vi "NF WF1973_74 TRAC Copy.vi"(5 "Name(USERNAME)":string="USERNAME", 7 "Memory No.(0)":i32 min=0 max=128 step=1, 8 "error in (no error)":errorcluster caption="Error IN", 9 "Select Function(Sin)":i32(ring)=2 items=["Sinusoid", "Square", "Pulse", "Ramp", "USine", "CSine", "CFCSine", "ACSine", "SSine", "MCSine", "ONPSine", "OFPSine", "CONSine", "COFSine", "Gaussian", "Lorents", "Haversine", "HSPulse", "TPulse", "Sinc", "ERise", "EFall", "Solstep", "Doscillation", "OSurge", "PSurge", "TOffset", "HSEPulse", "BRRamp", "USER"], 10 "Ch?(Ch1)":bool, 11 "VISAsession":refnum<visa-resource-name>) -> (0 "error out":errorcluster caption="Error OUT", 3 "CopyVISAsession":refnum<visa-resource-name>)   [LabVIEW 2010]
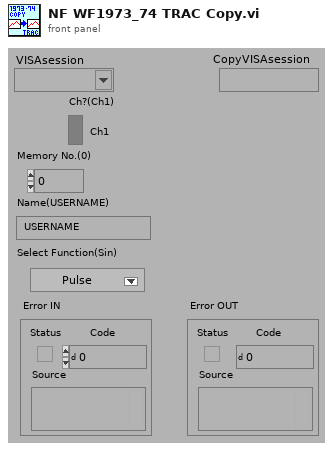
[diagram p1: front panel]
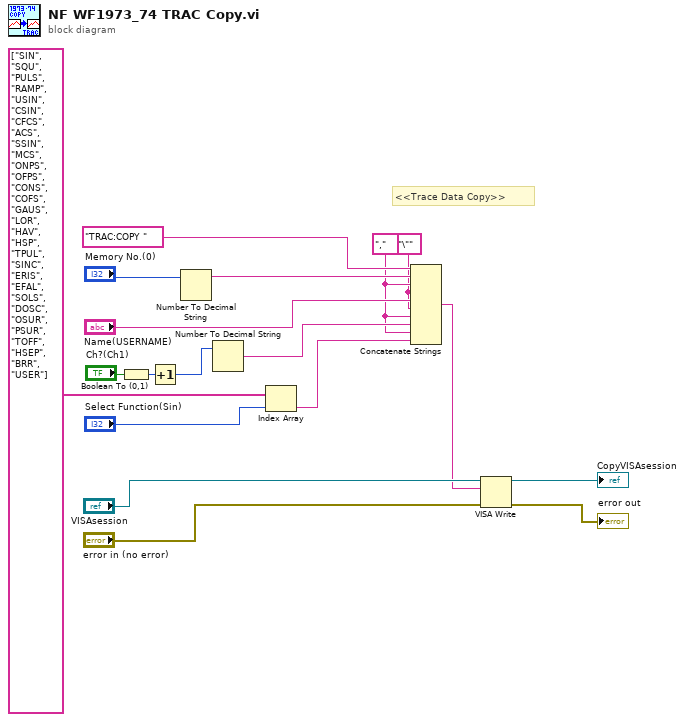
[diagram p0: block diagram]
diagram:
  w2 = "\""
  w5 = ","
  # "<<Trace Data Copy>>"
  n1 = Boolean To (0,1)(Boolean="Ch?(Ch1)") -> (0, 1=w8:i16)
  n2 = Increment(x=w8) -> (x+1=w4:i16)
  n3 = Number To Decimal String(number="Memory No.(0)") -> (decimal integer string=w11:string)  [unwired: 1 in]
  n4 = Number To Decimal String(number=w4) -> (decimal integer string=w7:string)  [unwired: 1 in]
  n5 = Index Array(array=string[] ["SIN", "SQU", "PULS", "RAMP", "USIN", "CSIN", "CFCS", "ACS", "SSIN", "MCS", "ONPS", "OFPS", "CONS", "COFS", "GAUS", "LOR", "HAV", "HSP", "TPUL", "SINC", "ERIS", "EFAL", "SOLS", "DOSC", "OSUR", "PSUR", "TOFF", "HSEP", "BRR", "USER"] ("配列"), index="Select Function(Sin)") -> (element=w6:string)
  n6 = Concatenate Strings("TRAC:COPY ", w11, w5, w2, "Name(USERNAME)", w2, w5, w7, w5, w6) -> (w3:string)
  n7 = VISA Write(VISA resource name="VISAsession", write buffer=w3, error in (no error)="error in (no error)") -> (VISA resource name out=→"CopyVISAsession":refnum<visa-resource-name>, error out=→"error out":errorcluster)  [unwired: 1 out]
